vi "rad_FPGA Bitfile deployment.vi"(8 "error in (no error)":errorcluster, 9 "Bitfile path":path, 10 "Resource Name":string, 11 "IP Address":string) -> (0 "error out":errorcluster)   [LabVIEW 2020]
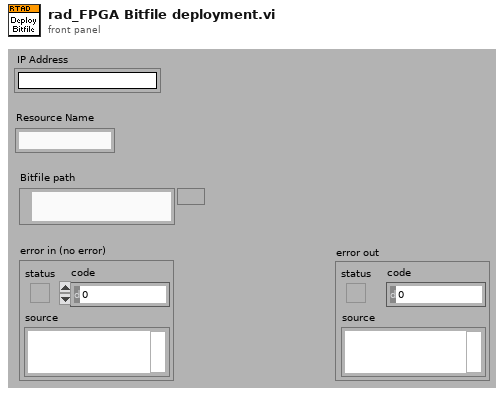
[diagram p1: front panel]
types:
  T1 = enum32{"Differential", "Referenced Single-Ended", "Nonreferenced Single-Ended"}
  T2 = enum32{"Do Not Autoload on Reset", "Autoload on Power-On Reset", "Autoload on Any Device Reset"}
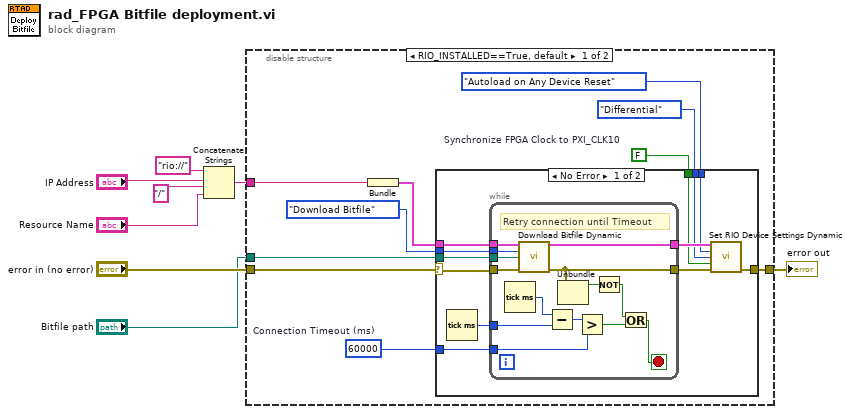
[diagram p0: block diagram]
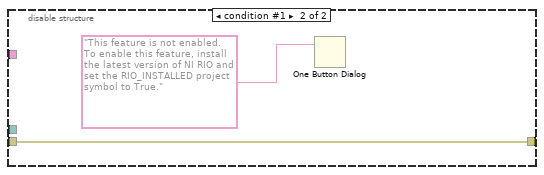
[diagram p3: hidden frame]
diagram:
  n1 = Concatenate Strings("rio://" ("string"), "IP Address", "/" ("string"), "Resource Name") -> (w5:string)
  n2 = disable-structure shown="RIO_INSTALLED==True, default" {
    disable-tunnel: w5 -> [w9 _]
    disable-tunnel: "error in (no error)" -> [w10 w47]
    disable-tunnel: [w18 w47] -> w3
    disable-tunnel: "Bitfile path" -> [w15 _]
    frame condition #0 (active) {
      w11 = u32 60000  # Connection Timeout (ms)
      w12 = FALSE  # Synchronize FPGA Clock to PXI_CLK10
      n3 = Bundle(w9) -> (w17:cluster{string})  [unwired: 1 in]
      n4 = case shown="No Error" w10 {
        selector: w10 -> [w19 w45]
        tunnel: [w30 w45] -> w18
        tunnel: w17 -> [w29 _]
        tunnel: enum16{"Erase Flash", "Download Bitfile"}."Download Bitfile" ("Operation (0:Erase Flash)") -> [w28 _]
        tunnel: w15 -> [w27 _]
        tunnel: T2."Autoload on Any Device Reset" ("FPGA AutoLoad Mode") -> [w25 _]
        tunnel: T1."Differential" ("Analog Input Mode") -> [w24 _]
        tunnel: w12 -> [w23 _]
        tunnel: w11 -> [w21 _]
        frame No Error {
          n5 = Tick Count (ms)() -> (millisecond timer value=w20:u32)
          n6 = while {
            tunnel: w19 -> [w44]
            tunnel: w29 -> [w43]
            tunnel: w28 -> [w42]
            tunnel: w27 -> [w41]
            tunnel: [w40] -> w26
            tunnel: [w35] -> w22
            tunnel: w20 -> [w38]
            tunnel: w21 -> [w36]
            stop <- w31 stop-if-true
            # "Retry connection until Timeout"
            n7 = Tick Count (ms)() -> (millisecond timer value=w39:u32)
            n8 = call "Download Bitfile Dynamic.vi"("Target Info"=w43, "Operation (0:Erase Flash)"=w42, "Bitfile Path"=w41, "Error In"=w44) -> ("Target Info Out"=w40:cluster{"FPGA Target Resource":string}, "Error Out"=w35:errorcluster)  [unwired: 10 in]
            n9 = Subtract(x=w39, y=w38) -> (x-y=w37:u32)
            n10 = Unbundle(w35) -> ("status"=w34:bool)  [unwired: 2 out]
            n11 = Greater?(x=w37, y=w36) -> (0:w32:bool)
            n12 = Not(x=w34) -> (.not. x?=w33:bool)
            n13 = Or(x=w33, y=w32) -> (x .or. y?=w31:bool)
          }
          n14 = call "Set RIO Device Settings Dynamic.vi"("Target Info"=w26, "FPGA AutoLoad Mode"=w25, "Analog Input Mode"=w24, "Synchronize FPGA Clock to PXI_CLK10"=w23, "Error In"=w22) -> ("Error Out"=w30:errorcluster)  [unwired: 9 in, 1 out]
        }
        frame Error {
        }
      }
    }
    frame condition #1 {
      n15 = One Button Dialog(message="This feature is not enabled.  To enable this feature, install the latest version of NI RIO and set the RIO_INSTALLED project symbol to True.") -> ()  [unwired: 1 in, 1 out]
    }
  }
  "error out" <- w3
